vi "Insert Indicators to [8,8] Array.vi"(7 "indicators":refnum<vi>[](array[refnum]), 9 "2-D controls references":refnum<vi>[][](array[refnum]), 11 "controls":refnum<vi>[](array[refnum])) -> (1 "2-D controls references out":refnum<vi>[][](array[refnum]))   [LabVIEW 2018, in "NISAST VI Scripting.lvlib" / "VI.lvlib" / "Front Panel.lvlib"]
uses:
  Front Panel.lvlib
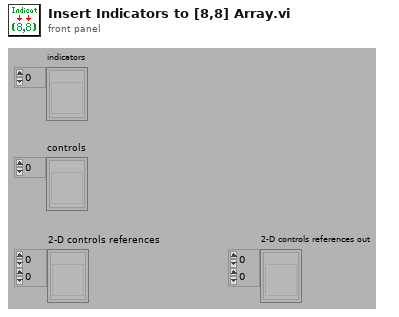
[diagram p1: front panel]
types:
  T1 = cluster{"Index (row)":i32, "Disabled Index (col)":i32}[]
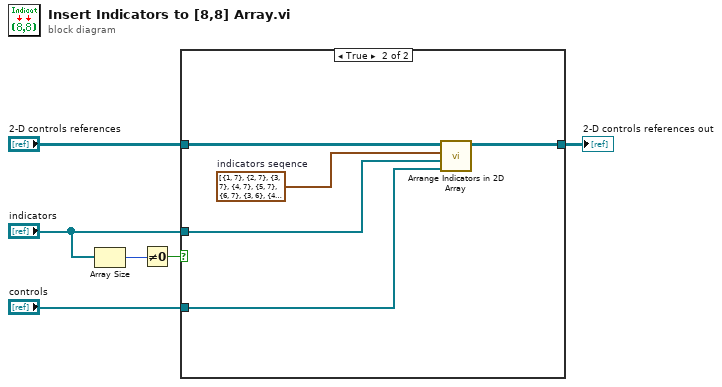
[diagram p0: block diagram]
diagram:
  n1 = Array Size(array="indicators") -> (size(s)=w4:i32)
  n2 = Not Equal To 0?(x=w4) -> (x != 0?=w3:bool)
  n3 = case shown="True" w3 {
    tunnel: "2-D controls references" -> [w7 w12]
    tunnel: [w7 w11] -> w2
    tunnel: "indicators" -> [_ w9]
    tunnel: "controls" -> [_ w8]
    frame False {
    }
    frame True {
      w10 = T1 [{"Index (row)"=1, "Disabled Index (col)"=7}, {"Index (row)"=2, "Disabled Index (col)"=7}, {"Index (row)"=3, "Disabled Index (col)"=7}, {"Index (row)"=4, "Disabled Index (col)"=7}, {"Index (row)"=5, "Disabled Index (col)"=7}, {"Index (row)"=6, "Disabled Index (col)"=7}, {"Index (row)"=3, "Disabled Index (col)"=6}, {"Index (row)"=4, "Disabled Index (col)"=6}, {"Index (row)"=3, "Disabled Index (col)"=5}, {"Index (row)"=4, "Disabled Index (col)"=5}, {"Index (row)"=3, "Disabled Index (col)"=4}, {"Index (row)"=4, "Disabled Index (col)"=4}, {"Index (row)"=3, "Disabled Index (col)"=3}, {"Index (row)"=4, "Disabled Index (col)"=3}, {"Index (row)"=3, "Disabled Index (col)"=2}, {"Index (row)"=4, "Disabled Index (col)"=2}, {"Index (row)"=3, "Disabled Index (col)"=1}, {"Index (row)"=4, "Disabled Index (col)"=1}, {"Index (row)"=6, "Disabled Index (col)"=0}, {"Index (row)"=5, "Disabled Index (col)"=0}, {"Index (row)"=4, "Disabled Index (col)"=0}, {"Index (row)"=3, "Disabled Index (col)"=0}, {"Index (row)"=2, "Disabled Index (col)"=0}, {"Index (row)"=1, "Disabled Index (col)"=0}]  # indicators seqence
      n4 = call "Arrange Indicators in 2D Array.vi"("controls"=w8, "indicators"=w9, "indicators seqence"=w10, "2-D references array"=w12) -> ("2-D references array out"=w11:refnum<vi>[][])  [unwired: 7 out]
    }
  }
  "2-D controls references out" <- w2
